vi "test TCX read (installed 71).vi"() -> ()   [LabVIEW 2011] (continued)
3:18:19Z</Time><Position><LatitudeDegrees>35.875570</LatitudeDegrees><LongitudeDegrees>-78.927722</LongitudeDegrees></Position><AltitudeMeters>68.872</AltitudeMeters><DistanceMeters>18272.553</DistanceMeters><Cadence>74</Cadence><Extensions><TPX xmlns=\"http://www.garmin.com/xmlschemas/ActivityExtension/v2\"><Watts>164</Watts></TPX></Extensions></Trackpoint><Trackpoint><Time>2008-03-03T23:18:20Z</Time><Position><LatitudeDegrees>35.875575</LatitudeDegrees><LongitudeDegrees>-78.927802</LongitudeDegrees></Position><AltitudeMeters>68.391</AltitudeMeters><DistanceMeters>18279.793</DistanceMeters><Cadence>73</Cadence><Extensions><TPX xmlns=\"http://www.garmin.com/xmlschemas/ActivityExtension/v2\"><Watts>157</Watts></TPX></Extensions></Trackpoint><Trackpoint><Time>2008-03-03T23:18:21Z</Time><Position><LatitudeDegrees>35.875583</LatitudeDegrees><LongitudeDegrees>-78.927883</LongitudeDegrees></Position><AltitudeMeters>68.872</AltitudeMeters><DistanceMeters>18287.141</DistanceMeters><Cadence>68</Cadence><Extensions><TPX xmlns=\"http://www.garmin.com/xmlschemas/ActivityExtension/v2\"><Watts>132</Watts></TPX></Extensions></Trackpoint><Trackpoint><Time>2008-03-03T23:18:22Z</Time><Position><LatitudeDegrees>35.875591</LatitudeDegrees><LongitudeDegrees>-78.927967</LongitudeDegrees></Position><AltitudeMeters>68.391</AltitudeMeters><DistanceMeters>18294.795</DistanceMeters><Cadence>69</Cadence><Extensions><TPX xmlns=\"http://www.garmin.com/xmlschemas/ActivityExtension/v2\"><Watts>106</Watts></TPX></Extensions></Trackpoint><Trackpoint><Time>2008-03-03T23:18:23Z</Time><Position><LatitudeDegrees>35.875599</LatitudeDegrees><LongitudeDegrees>-78.928051</LongitudeDegrees></Position><AltitudeMeters>68.872</AltitudeMeters><DistanceMeters>18302.459</DistanceMeters><Cadence>70</Cadence><Extensions><TPX xmlns=\"http://www.garmin.com/xmlschemas/ActivityExtension/v2\"><Watts>105</Watts></TPX></Extensions></Trackpoint><Trackpoint><Time>2008-03-03T23:18:24Z</Time><Position><LatitudeDegrees>35.875607</LatitudeDegrees><LongitudeDegrees>-78.928138</LongitudeDegrees></Position><AltitudeMeters>68.872</AltitudeMeters><DistanceMeters>18310.340</DistanceMeters><Cadence>71</Cadence><Extensions><TPX xmlns=\"http://www.garmin.com/xmlschemas/ActivityExtension/v2\"><Watts>95</Watts></TPX></Extensions></Trackpoint><Trackpoint><Time>2008-03-03T23:18:25Z</Time><Position><LatitudeDegrees>35.875615</LatitudeDegrees><LongitudeDegrees>-78.928227</LongitudeDegrees></Position><AltitudeMeters>68.391</AltitudeMeters><DistanceMeters>18318.404</DistanceMeters><Cadence>73</Cadence><Extensions><TPX xmlns=\"http://www.garmin.com/xmlschemas/ActivityExtension/v2\"><Watts>74</Watts></TPX></Extensions></Trackpoint><Trackpoint><Time>2008-03-03T23:18:26Z</Time><Position><LatitudeDegrees>35.875623</LatitudeDegrees><LongitudeDegrees>-78.928316</LongitudeDegrees></Position><AltitudeMeters>68.391</AltitudeMeters><DistanceMeters>18326.637</DistanceMeters><Cadence>75</Cadence><Extensions><TPX xmlns=\"http://www.garmin.com/xmlschemas/ActivityExtension/v2\"><Watts>63</Watts></TPX></Extensions></Trackpoint><Trackpoint><Time>2008-03-03T23:18:27Z</Time><Position><LatitudeDegrees>35.875631</LatitudeDegrees><LongitudeDegrees>-78.928409</LongitudeDegrees></Position><AltitudeMeters>67.910</AltitudeMeters><DistanceMeters>18334.977</DistanceMeters><Cadence>75</Cadence><Extensions><TPX xmlns=\"http://www.garmin.com/xmlschemas/ActivityExtension/v2\"><Watts>64</Watts></TPX></Extensions></Trackpoint><Trackpoint><Time>2008-03-03T23:18:28Z</Time><Position><LatitudeDegrees>35.875640</LatitudeDegrees><LongitudeDegrees>-78.928504</LongitudeDegrees></Position><AltitudeMeters>67.910</AltitudeMeters><DistanceMeters>18343.660</DistanceMeters><Cadence>81</Cadence><Extensions><TPX xmlns=\"http://www.garmin.com/xmlschemas/ActivityExtension/v2\"><Watts>53</Watts></TPX></Extensions></Trackpoint><Trackpoint><Time>2008-03-03T23:18:29Z</Time><Position><LatitudeDegrees>35.875651</LatitudeDegrees><LongitudeDegrees>-78.928603</LongitudeDegrees></Position><AltitudeMeters>67.910</AltitudeMeters><DistanceMeters>18352.664</DistanceMeters><Cadence>83</Cadence><Extensions><TPX xmlns=\"http://www.garmin.com/xmlschemas/ActivityExtension/v2\"><Watts>51</Watts></TPX></Extensions></Trackpoint><Trackpoint><Time>2008-03-03T23:18:30Z</Time><Position><LatitudeDegrees>35.875663</LatitudeDegrees><LongitudeDegrees>-78.928704</LongitudeDegrees></Position><AltitudeMeters>67.430</AltitudeMeters><DistanceMeters>18361.902</DistanceMeters><Cadence>85</Cadence><Extensions><TPX xmlns=\"http://www.garmin.com/xmlschemas/ActivityExtension/v2\"><Watts>48</Watts></TPX></Extensions></Trackpoint><Trackpoint><Time>2008-03-03T23:18:31Z</Time><Position><LatitudeDegrees>35.875675</LatitudeDegrees><LongitudeDegrees>-78.928807</LongitudeDegrees></Position><AltitudeMeters>66.949</AltitudeMeters><DistanceMeters>18371.299</DistanceMeters><Cadence>87</Cadence><Extensions><TPX xmlns=\"http://www.garmin.com/xmlschemas/ActivityExtension/v2\"><Watts>48</Watts></TPX></Extensions></Trackpoint><Trackpoint><Time>2008-03-03T23:18:32Z</Time><Position><LatitudeDegrees>35.875686</LatitudeDegrees><LongitudeDegrees>-78.928912</LongitudeDegrees></Position><AltitudeMeters>66.468</AltitudeMeters><DistanceMeters>18380.938</DistanceMeters><Cadence>90</Cadence><Extensions><TPX xmlns=\"http://www.garmin.com/xmlschemas/ActivityExtension/v2\"><Watts>50</Watts></TPX></Extensions></Trackpoint><Trackpoint><Time>2008-03-03T23:18:33Z</Time><Position><LatitudeDegrees>35.875695</LatitudeDegrees><LongitudeDegrees>-78.929021</LongitudeDegrees></Position><AltitudeMeters>65.988</AltitudeMeters><DistanceMeters>18390.785</DistanceMeters><Cadence>91</Cadence><Extensions><TPX xmlns=\"http://www.garmin.com/xmlschemas/ActivityExtension/v2\"><Watts>58</Watts></TPX></Extensions></Trackpoint><Trackpoint><Time>2008-03-03T23:18:34Z</Time><Position><LatitudeDegrees>35.875703</LatitudeDegrees><LongitudeDegrees>-78.929130</LongitudeDegrees></Position><AltitudeMeters>65.988</AltitudeMeters><DistanceMeters>18400.648</DistanceMeters><Cadence>91</Cadence><Extensions><TPX xmlns=\"http://www.garmin.com/xmlschemas/ActivityExtension/v2\"><Watts>66</Watts></TPX></Extensions></Trackpoint><Trackpoint><Time>2008-03-03T23:18:35Z</Time><Position><LatitudeDegrees>35.875709</LatitudeDegrees><LongitudeDegrees>-78.929239</LongitudeDegrees></Position><AltitudeMeters>65.988</AltitudeMeters><DistanceMeters>18410.574</DistanceMeters><Cadence>91</Cadence><Extensions><TPX xmlns=\"http://www.garmin.com/xmlschemas/ActivityExtension/v2\"><Watts>67</Watts></TPX></Extensions></Trackpoint><Trackpoint><Time>2008-03-03T23:18:36Z</Time><Position><LatitudeDegrees>35.875717</LatitudeDegrees><LongitudeDegrees>-78.929349</LongitudeDegrees></Position><AltitudeMeters>65.988</AltitudeMeters><DistanceMeters>18420.459</DistanceMeters><Cadence>91</Cadence><Extensions><TPX xmlns=\"http://www.garmin.com/xmlschemas/ActivityExtension/v2\"><Watts>71</Watts></TPX></Extensions></Trackpoint><Trackpoint><Time>2008-03-03T23:18:37Z</Time><Position><LatitudeDegrees>35.875727</LatitudeDegrees><LongitudeDegrees>-78.929458</LongitudeDegrees></Position><AltitudeMeters>65.988</AltitudeMeters><DistanceMeters>18430.391</DistanceMeters><Cadence>91</Cadence><Extensions><TPX xmlns=\"http://www.garmin.com/xmlschemas/ActivityExtension/v2\"><Watts>71</Watts></TPX></Extensions></Trackpoint><Trackpoint><Time>2008-03-03T23:18:38Z</Time><Position><LatitudeDegrees>35.875738</LatitudeDegrees><LongitudeDegrees>-78.929565</LongitudeDegrees></Position><AltitudeMeters>65.988</AltitudeMeters><DistanceMeters>18440.133</DistanceMeters><Cadence>90</Cadence><Extensions><TPX xmlns=\"http://www.garmin.com/xmlschemas/ActivityExtension/v2\"><Watts>78</Watts></TPX></Extensions></Trackpoint><Trackpoint><Time>2008-03-03T23:18:39Z</Time><Position><LatitudeDegrees>35.875745</LatitudeDegrees><LongitudeDegrees>-78.929673</LongitudeDegrees></Position><AltitudeMeters>65.507</AltitudeMeters><DistanceMeters>18449.887</DistanceMeters><Cadence>90</Cadence><Extensions><TPX xmlns=\"http://www.garmin.com/xmlschemas/ActivityExtension/v2\"><Watts>79</Watts></TPX></Extensions></Trackpoint><Trackpoint><Time>2008-03-03T23:18:40Z</Time><Position><LatitudeDegrees>35.875749</LatitudeDegrees><LongitudeDegrees>-78.929779</LongitudeDegrees></Position><AltitudeMeters>65.988</AltitudeMeters><DistanceMeters>18459.521</DistanceMeters><Cadence>89</Cadence><Extensions><TPX xmlns=\"http://www.garmin.com/xmlschemas/ActivityExtension/v2\"><Watts>101</Watts></TPX></Extensions></Trackpoint><Trackpoint><Time>2008-03-03T23:18:41Z</Time><Position><LatitudeDegrees>35.875754</LatitudeDegrees><LongitudeDegrees>-78.929886</LongitudeDegrees></Position><AltitudeMeters>65.988</AltitudeMeters><DistanceMeters>18469.232</DistanceMeters><Cadence>88</Cadence><Extensions><TPX xmlns=\"http://www.garmin.com/xmlschemas/ActivityExtension/v2\"><Watts>106</Watts></TPX></Extensions></Trackpoint><Trackpoint><Time>2008-03-03T23:18:42Z</Time><Position><LatitudeDegrees>35.875758</LatitudeDegrees><LongitudeDegrees>-78.929991</LongitudeDegrees></Position><AltitudeMeters>65.507</AltitudeMeters><DistanceMeters>18478.709</DistanceMeters><Cadence>87</Cadence><Extensions><TPX xmlns=\"http://www.garmin.com/xmlschemas/ActivityExtension/v2\"><Watts>106</Watts></TPX></Extensions></Trackpoint><Trackpoint><Time>2008-03-03T23:18:43Z</Time><Position><LatitudeDegrees>35.875761</LatitudeDegrees><LongitudeDegrees>-78.930095</LongitudeDegrees></Position><AltitudeMeters>65.507</AltitudeMeters><DistanceMeters>18488.055</DistanceMeters><Cadence>86</Cadence><Extensions><TPX xmlns=\"http://www.garmin.com/xmlschemas/ActivityExtension/v2\"><Watts>113</Watts></TPX></Extensions></Trackpoint><Trackpoint><Time>2008-03-03T23:18:44Z</Time><Position><LatitudeDegrees>35.875764</LatitudeDegrees><LongitudeDegrees>-78.930200</LongitudeDegrees></Position><AltitudeMeters>65.507</AltitudeMeters><DistanceMeters>18497.482</DistanceMeters><Cadence>86</Cadence><Extensions><TPX xmlns=\"http://www.garmin.com/xmlschemas/ActivityExtension/v2\"><Watts>112</Watts></TPX></Extensions></Trackpoint><Trackpoint><Time>2008-03-03T23:18:45Z</Time><Position><LatitudeDegrees>35.875767</LatitudeDegrees><LongitudeDegrees>-78.930301</LongitudeDegrees></Position><AltitudeMeters>65.507</AltitudeMeters><DistanceMeters>18506.688</DistanceMeters><Cadence>85</Cadence><Extensions><TPX xmlns=\"http://www.garmin.com/xmlschemas/ActivityExtension/v2\"><Watts>118</Watts></TPX></Extensions></Trackpoint><Trackpoint><Time>2008-03-03T23:18:46Z</Time><Position><LatitudeDegrees>35.875770</LatitudeDegrees><LongitudeDegrees>-78.930402</LongitudeDegrees></Position><AltitudeMeters>65.988</AltitudeMeters><DistanceMeters>18515.820</DistanceMeters><Cadence>84</Cadence><Extensions><TPX xmlns=\"http://www.garmin.com/xmlschemas/ActivityExtension/v2\"><Watts>133</Watts></TPX></Extensions></Trackpoint><Trackpoint><Time>2008-03-03T23:18:47Z</Time><Position><LatitudeDegrees>35.875772</LatitudeDegrees><LongitudeDegrees>-78.930502</LongitudeDegrees></Position><AltitudeMeters>65.988</AltitudeMeters><DistanceMeters>18524.832</DistanceMeters><Cadence>84</Cadence><Extensions><TPX xmlns=\"http://www.garmin.com/xmlschemas/ActivityExtension/v2\"><Watts>159</Watts></TPX></Extensions></Trackpoint><Trackpoint><Time>2008-03-03T23:18:48Z</Time><Position><LatitudeDegrees>35.875773</LatitudeDegrees><LongitudeDegrees>-78.930602</LongitudeDegrees></Position><AltitudeMeters>65.988</AltitudeMeters><DistanceMeters>18533.852</DistanceMeters><Cadence>83</Cadence><Extensions><TPX xmlns=\"http://www.garmin.com/xmlschemas/ActivityExtension/v2\"><Watts>166</Watts></TPX></Extensions></Trackpoint><Trackpoint><Time>2008-03-03T23:18:49Z</Time><Position><LatitudeDegrees>35.875777</LatitudeDegrees><LongitudeDegrees>-78.930701</LongitudeDegrees></Position><AltitudeMeters>65.988</AltitudeMeters><DistanceMeters>18542.797</DistanceMeters><Cadence>83</Cadence><Extensions><TPX xmlns=\"http://www.garmin.com/xmlschemas/ActivityExtension/v2\"><Watts>168</Watts></TPX></Extensions></Trackpoint><Trackpoint><Time>2008-03-03T23:18:50Z</Time><Position><LatitudeDegrees>35.875781</LatitudeDegrees><LongitudeDegrees>-78.930800</LongitudeDegrees></Position><AltitudeMeters>66.468</AltitudeMeters><DistanceMeters>18551.742</DistanceMeters><Cadence>82</Cadence><Extensions><TPX xmlns=\"http://www.garmin.com/xmlschemas/ActivityExtension/v2\"><Watts>183</Watts></TPX></Extensions></Trackpoint><Trackpoint><Time>2008-03-03T23:18:51Z</Time><Position><LatitudeDegrees>35.875783</LatitudeDegrees><LongitudeDegrees>-78.930898</LongitudeDegrees></Position><AltitudeMeters>65.988</AltitudeMeters><DistanceMeters>18560.613</DistanceMeters><Cadence>81</Cadence><Extensions><TPX xmlns=\"http://www.garmin.com/xmlschemas/ActivityExtension/v2\"><Watts>177</Watts></TPX></Extensions></Trackpoint><Trackpoint><Time>2008-03-03T23:18:52Z</Time><Position><LatitudeDegrees>35.875787</LatitudeDegrees><LongitudeDegrees>-78.930996</LongitudeDegrees></Position><AltitudeMeters>65.988</AltitudeMeters><DistanceMeters>18569.484</DistanceMeters><Cadence>80</Cadence><Extensions><TPX xmlns=\"http://www.garmin.com/xmlschemas/ActivityExtension/v2\"><Watts>171</Watts></TPX></Extensions></Trackpoint><Trackpoint><Time>2008-03-03T23:18:53Z</Time><Position><LatitudeDegrees>35.875790</LatitudeDegrees><LongitudeDegrees>-78.931093</LongitudeDegrees></Position><AltitudeMeters>65.988</AltitudeMeters><DistanceMeters>18578.180</DistanceMeters><Cadence>79</Cadence><Extensions><TPX xmlns=\"http://www.garmin.com/xmlschemas/ActivityExtension/v2\"><Watts>163</Watts></TPX></Extensions></Trackpoint><Trackpoint><Time>2008-03-03T23:18:54Z</Time><Position><LatitudeDegrees>35.875789</LatitudeDegrees><LongitudeDegrees>-78.931187</LongitudeDegrees></Position><AltitudeMeters>65.988</AltitudeMeters><DistanceMeters>18586.668</DistanceMeters><Cadence>79</Cadence><Extensions><TPX xmlns=\"http://www.garmin.com/xmlschemas/ActivityExtension/v2\"><Watts>162</Watts></TPX></Extensions></Trackpoint><Trackpoint><Time>2008-03-03T23:18:55Z</Time><Position><LatitudeDegrees>35.875786</LatitudeDegrees><LongitudeDegrees>-78.931280</LongitudeDegrees></Position><AltitudeMeters>65.988</AltitudeMeters><DistanceMeters>18595.109</DistanceMeters><Cadence>78</Cadence><Extensions><TPX xmlns=\"http://www.garmin.com/xmlschemas/ActivityExtension/v2\"><Watts>163</Watts></TPX></Extensions></Trackpoint><Trackpoint><Time>2008-03-03T23:18:56Z</Time><Position><LatitudeDegrees>35.875781</LatitudeDegrees><LongitudeDegrees>-78.931372</LongitudeDegrees></Position><AltitudeMeters>66.468</AltitudeMeters><DistanceMeters>18603.369</DistanceMeters><Cadence>77</Cadence><Extensions><TPX xmlns=\"http://www.garmin.com/xmlschemas/ActivityExtension/v2\"><Watts>164</Watts></TPX></Extensions></Trackpoint><Trackpoint><Time>2008-03-03T23:18:57Z</Time><Position><LatitudeDegrees>35.875773</LatitudeDegrees><LongitudeDegrees>-78.931461</LongitudeDegrees></Position><AltitudeMeters>66.468</AltitudeMeters><DistanceMeters>18611.516</DistanceMeters><Cadence>75</Cadence><Extensions><TPX xmlns=\"http://www.garmin.com/xmlschemas/ActivityExtension/v2\"><Watts>157</Watts></TPX></Extensions></Trackpoint><Trackpoint><Time>2008-03-03T23:18:58Z</Time><Position><LatitudeDegrees>35.875762</LatitudeDegrees><LongitudeDegrees>-78.931550</LongitudeDegrees></Position><AltitudeMeters>66.468</AltitudeMeters><DistanceMeters>18619.531</DistanceMeters><Cadence>73</Cadence><Extensions><TPX xmlns=\"http://www.garmin.com/xmlschemas/ActivityExtension/v2\"><Watts>164</Watts></TPX></Extensions></Trackpoint><Trackpoint><Time>2008-03-03T23:18:59Z</Time><Position><LatitudeDegrees>35.875749</LatitudeDegrees><LongitudeDegrees>-78.931636</LongitudeDegrees></Position><AltitudeMeters>66.949</AltitudeMeters><DistanceMeters>18627.453</DistanceMeters><Cadence>73</Cadence><Extensions><TPX xmlns=\"http://www.garmin.com/xmlschemas/ActivityExtension/v2\"><Watts>168</Watts></TPX></Extensions></Trackpoint><Trackpoint><Time>2008-03-03T23:19:00Z</Time><Position><LatitudeDegrees>35.875735</LatitudeDegrees><LongitudeDegrees>-78.931720</LongitudeDegrees></Position><AltitudeMeters>67.430</AltitudeMeters><DistanceMeters>18635.238</DistanceMeters><Cadence>71</Cadence><Extensions><TPX xmlns=\"http://www.garmin.com/xmlschemas/ActivityExtension/v2\"><Watts>181</Watts></TPX></Extensions></Trackpoint><Trackpoint><Time>2008-03-03T23:19:01Z</Time><Position><LatitudeDegrees>35.875721</LatitudeDegrees><LongitudeDegrees>-78.931803</LongitudeDegrees></Position><AltitudeMeters>67.430</AltitudeMeters><DistanceMeters>18642.844</DistanceMeters><Cadence>69</Cadence><Extensions><TPX xmlns=\"http://www.garmin.com/xmlschemas/ActivityExtension/v2\"><Watts>207</Watts></TPX></Extensions></Trackpoint><Trackpoint><Time>2008-03-03T23:19:02Z</Time><Position><LatitudeDegrees>35.875705</LatitudeDegrees><LongitudeDegrees>-78.931884</LongitudeDegrees></Position><AltitudeMeters>67.430</AltitudeMeters><DistanceMeters>18650.436</DistanceMeters><Cadence>70</Cadence><Extensions><TPX xmlns=\"http://www.garmin.com/xmlschemas/ActivityExtension/v2\"><Watts>205</Watts></TPX></Extensions></Trackpoint><Trackpoint><Time>2008-03-03T23:19:03Z</Time><Position><LatitudeDegrees>35.875691</LatitudeDegrees><LongitudeDegrees>-78.931962</LongitudeDegrees></Position><AltitudeMeters>67.910</AltitudeMeters><DistanceMeters>18657.533</DistanceMeters><Cadence>73</Cadence><Extensions><TPX xmlns=\"http://www.garmin.com/xmlschemas/ActivityExtension/v2\"><Watts>188</Watts></TPX></Extensions></Trackpoint><Trackpoint><Time>2008-03-03T23:19:04Z</Time><Position><LatitudeDegrees>35.875675</LatitudeDegrees><LongitudeDegrees>-78.932036</LongitudeDegrees></Position><AltitudeMeters>68.391</AltitudeMeters><DistanceMeters>18664.455</DistanceMeters><Cadence>73</Cadence><Extensions><TPX xmlns=\"http://www.garmin.com/xmlschemas/ActivityExtension/v2\"><Watts>185</Watts></TPX></Extensions></Trackpoint><Trackpoint><Time>2008-03-03T23:19:05Z</Time><Position><LatitudeDegrees>35.875659</LatitudeDegrees><LongitudeDegrees>-78.932107</LongitudeDegrees></Position><AltitudeMeters>68.391</AltitudeMeters><DistanceMeters>18671.105</DistanceMeters><Cadence>76</Cadence><Extensions><TPX xmlns=\"http://www.garmin.com/xmlschemas/ActivityExtension/v2\"><Watts>174</Watts></TPX></Extensions></Trackpoint><Trackpoint><Time>2008-03-03T23:19:06Z</Time><Position><LatitudeDegrees>35.875644</LatitudeDegrees><LongitudeDegrees>-78.932177</LongitudeDegrees></Position><AltitudeMeters>68.872</AltitudeMeters><DistanceMeters>18677.600</DistanceMeters><Cadence>78</Cadence><Extensions><TPX xmlns=\"http://www.garmin.com/xmlschemas/ActivityExtension/v2\"><Watts>173</Watts></TPX></Extensions></Trackpoint><Trackpoint><Time>2008-03-03T23:19:07Z</Time><Position><LatitudeDegrees>35.875631</LatitudeDegrees><LongitudeDegrees>-78.932247</LongitudeDegrees></Position><AltitudeMeters>69.352</AltitudeMeters><DistanceMeters>18684.131</DistanceMeters><Cadence>79</Cadence><Extensions><TPX xmlns=\"http://www.garmin.com/xmlschemas/ActivityExtension/v2\"><Watts>237</Watts></TPX></Extensions></Trackpoint><Trackpoint><Time>2008-03-03T23:19:08Z</Time><Position><LatitudeDegrees>35.875617</LatitudeDegrees><LongitudeDegrees>-78.932317</LongitudeDegrees></Position><AltitudeMeters>69.352</AltitudeMeters><DistanceMeters>18690.664</DistanceMeters><Cadence>79</Cadence><Extensions><TPX xmlns=\"http://www.garmin.com/xmlschemas/ActivityExtension/v2\"><Watts>338</Watts></TPX></Extensions></Trackpoint><Trackpoint><Time>2008-03-03T23:19:09Z</Time><Position><LatitudeDegrees>35.875603</LatitudeDegrees><LongitudeDegrees>-78.932388</LongitudeDegrees></Position><AltitudeMeters>69.833</AltitudeMeters><DistanceMeters>18697.219</DistanceMeters><Cadence>79</Cadence><Extensions><TPX xmlns=\"http://www.garmin.com/xmlschemas/ActivityExtension/v2\"><Watts>373</Watts></TPX></Extensions></Trackpoint><Trackpoint><Time>2008-03-03T23:19:10Z</Time><Position><LatitudeDegrees>35.875589</LatitudeDegrees><LongitudeDegrees>-78.932458</LongitudeDegrees></Position><AltitudeMeters>70.313</AltitudeMeters><DistanceMeters>18703.715</DistanceMeters><Cadence>78</Cadence><Extensions><TPX xmlns=\"http://www.garmin.com/xmlschemas/ActivityExtension/v2\"><Watts>371</Watts></TPX></Extensions></Trackpoint><Trackpoint><Time>2008-03-03T23:19:11Z</Time><Position><LatitudeDegrees>35.875575</LatitudeDegrees><LongitudeDegrees>-78.932527</LongitudeDegrees></Position><AltitudeMeters>70.794</AltitudeMeters><DistanceMeters>18710.178</DistanceMeters><Cadence>78</Cadence><Extensions><TPX xmlns=\"http://www.garmin.com/xmlschemas/ActivityExtension/v2\"><Watts>387</Watts></TPX></Extensions></Trackpoint><Trackpoint><Time>2008-03-03T23:19:12Z</Time><Position><LatitudeDegrees>35.875562</LatitudeDegrees><LongitudeDegrees>-78.932597</LongitudeDegrees></Position><AltitudeMeters>71.275</AltitudeMeters><DistanceMeters>18716.688</DistanceMeters><Cadence>79</Cadence><Extensions><TPX xmlns=\"http://www.garmin.com/xmlschemas/ActivityExtension/v2\"><Watts>457</Watts></TPX></Extensions></Trackpoint><Trackpoint><Time>2008-03-03T23:19:13Z</Time><Position><LatitudeDegrees>35.875548</LatitudeDegrees><LongitudeDegrees>-78.932668</LongitudeDegrees></Position><AltitudeMeters>71.755</AltitudeMeters><DistanceMeters>18723.232</DistanceMeters><Cadence>79</Cadence><Extensions><TPX xmlns=\"http://www.garmin.com/xmlschemas/ActivityExtension/v2\"><Watts>465</Watts></TPX></Extensions></Trackpoint><Trackpoint><Time>2008-03-03T23:19:14Z</Time><Position><LatitudeDegrees>35.875533</LatitudeDegrees><LongitudeDegrees>-78.932738</LongitudeDegrees></Position><AltitudeMeters>71.755</AltitudeMeters><DistanceMeters>18729.775</DistanceMeters><Cadence>79</Cadence><Extensions><TPX xmlns=\"http://www.garmin.com/xmlschemas/ActivityExtension/v2\"><Watts>467</Watts></TPX></Extensions></Trackpoint><Trackpoint><Time>2008-03-03T23:19:15Z</Time><Position><LatitudeDegrees>35.875519</LatitudeDegrees><LongitudeDegrees>-78.932808</LongitudeDegrees></Position><AltitudeMeters>72.236</AltitudeMeters><DistanceMeters>18736.256</DistanceMeters><Cadence>78</Cadence><Extensions><TPX xmlns=\"http://www.garmin.com/xmlschemas/ActivityExtension/v2\"><Watts>452</Watts></TPX></Extensions></Trackpoint><Trackpoint><Time>2008-03-03T23:19:16Z</Time><Position><LatitudeDegrees>35.875505</LatitudeDegrees><LongitudeDegrees>-78.932876</LongitudeDegrees></Position><AltitudeMeters>72.717</AltitudeMeters><DistanceMeters>18742.592</DistanceMeters><Cadence>78</Cadence><Extensions><TPX xmlns=\"http://www.garmin.com/xmlschemas/ActivityExtension/v2\"><Watts>448</Watts></TPX></Extensions></Trackpoint><Trackpoint><Time>2008-03-03T23:19:17Z</Time><Position><LatitudeDegrees>35.875492</LatitudeDegrees><LongitudeDegrees>-78.932942</LongitudeDegrees></Position><AltitudeMeters>73.198</AltitudeMeters><DistanceMeters>18748.783</DistanceMeters><Cadence>74</Cadence><Extensions><TPX xmlns=\"http://www.garmin.com/xmlschemas/ActivityExtension/v2\"><Watts>451</Watts></TPX></Extensions></Trackpoint><Trackpoint><Time>2008-03-03T23:19:18Z</Time><Position><LatitudeDegrees>35.875479</LatitudeDegrees><LongitudeDegrees>-78.933006</LongitudeDegrees></Position><AltitudeMeters>73.678</AltitudeMeters><DistanceMeters>18754.693</DistanceMeters><Cadence>71</Cadence><Extensions><TPX xmlns=\"http://www.garmin.com/xmlschemas/ActivityExtension/v2\"><Watts>459</Watts></TPX></Extensions></Trackpoint><Trackpoint><Time>2008-03-03T23:19:19Z</Time><Position><LatitudeDegrees>35.875466</LatitudeDegrees><LongitudeDegrees>-78.933069</LongitudeDegrees></Position><AltitudeMeters>73.678</AltitudeMeters><DistanceMeters>18760.582</DistanceMeters><Cadence>72</Cadence><Extensions><TPX xmlns=\"http://www.garmin.com/xmlschemas/ActivityExtension/v2\"><Watts>462</Watts></TPX></Extensions></Trackpoint><Trackpoint><Time>2008-03-03T23:19:20Z</Time><Position><LatitudeDegrees>35.875455</LatitudeDegrees><LongitudeDegrees>-78.933137</LongitudeDegrees></Position><AltitudeMeters>74.159</AltitudeMeters><DistanceMeters>18766.793</DistanceMeters><Cadence>73</Cadence><Extensions><TPX xmlns=\"http://www.garmin.com/xmlschemas/ActivityExtension/v2\"><Watts>525</Watts></TPX></Extensions></Trackpoint><Trackpoint><Time>2008-03-03T23:19:21Z</Time><Position><LatitudeDegrees>35.875441</LatitudeDegrees><LongitudeDegrees>-78.933206</LongitudeDegrees></Position><AltitudeMeters>74.640</AltitudeMeters><DistanceMeters>18773.268</DistanceMeters><Cadence>73</Cadence><Extensions><TPX xmlns=\"http://www.garmin.com/xmlschemas/ActivityExtension/v2\"><Watts>529</Watts></TPX></Extensions></Trackpoint><Trackpoint><Time>2008-03-03T23:19:22Z</Time><Position><LatitudeDegrees>35.875428</LatitudeDegrees><LongitudeDegrees>-78.933280</LongitudeDegrees></Position><AltitudeMeters>75.601</AltitudeMeters><DistanceMeters>18780.102</DistanceMeters><Cadence>83</Cadence><Extensions><TPX xmlns=\"http://www.garmin.com/xmlschemas/ActivityExtension/v2\"><Watts>697</Watts></TPX></Extensions></Trackpoint><Trackpoint><Time>2008-03-03T23:19:23Z</Time><Position><LatitudeDegrees>35.875415</LatitudeDegrees><LongitudeDegrees>-78.933356</LongitudeDegrees></Position><AltitudeMeters>75.601</AltitudeMeters><DistanceMeters>18787.135</DistanceMeters><Cadence>86</Cadence><Extensions><TPX xmlns=\"http://www.garmin.com/xmlschemas/ActivityExtension/v2\"><Watts>788</Watts></TPX></Extensions></Trackpoint><Trackpoint><Time>2008-03-03T23:19:24Z</Time><Position><LatitudeDegrees>35.875399</LatitudeDegrees><LongitudeDegrees>-78.933433</LongitudeDegrees></Position><AltitudeMeters>76.081</AltitudeMeters><DistanceMeters>18794.295</DistanceMeters><Cadence>86</Cadence><Extensions><TPX xmlns=\"http://www.garmin.com/xmlschemas/ActivityExtension/v2\"><Watts>782</Watts></TPX></Extensions></Trackpoint><Trackpoint><Time>2008-03-03T23:19:25Z</Time><Position><LatitudeDegrees>35.875377</LatitudeDegrees><LongitudeDegrees>-78.933509</LongitudeDegrees></Position><AltitudeMeters>77.043</AltitudeMeters><DistanceMeters>18801.568</DistanceMeters><Cadence>89</Cadence><Extensions><TPX xmlns=\"http://www.garmin.com/xmlschemas/ActivityExtension/v2\"><Watts>738</Watts></TPX></Extensions></Trackpoint><Trackpoint><Time>2008-03-03T23:19:26Z</Time><Position><LatitudeDegrees>35.875358</LatitudeDegrees><LongitudeDegrees>-78.933588</LongitudeDegrees></Position><AltitudeMeters>77.043</AltitudeMeters><DistanceMeters>18809.012</DistanceMeters><Cadence>91</Cadence><Extensions><TPX xmlns=\"http://www.garmin.com/xmlschemas/ActivityExtension/v2\"><Watts>743</Watts></TPX></Extensions></Trackpoint><Trackpoint><Time>2008-03-03T23:19:27Z</Time><Position><LatitudeDegrees>35.875341</LatitudeDegrees><LongitudeDegrees>-78.933670</LongitudeDegrees></Position><AltitudeMeters>77.523</AltitudeMeters><DistanceMeters>18816.676</DistanceMeters><Cadence>92</Cadence><Extensions><TPX xmlns=\"http://www.garmin.com/xmlschemas/ActivityExtension/v2\"><Watts>701</Watts></TPX></Extensions></Trackpoint><Trackpoint><Time>2008-03-03T23:19:28Z</Time><Position><LatitudeDegrees>35.875323</LatitudeDegrees><LongitudeDegrees>-78.933751</LongitudeDegrees></Position><AltitudeMeters>78.485</AltitudeMeters><DistanceMeters>18824.240</DistanceMeters><Cadence>91</Cadence><Extensions><TPX xmlns=\"http://www.garmin.com/xmlschemas/ActivityExtension/v2\"><Watts>567</Watts></TPX></Extensions></Trackpoint><Trackpoint><Time>2008-03-03T23:19:29Z</Time><Position><LatitudeDegrees>35.875308</LatitudeDegrees><LongitudeDegrees>-78.933832</LongitudeDegrees></Position><AltitudeMeters>79.446</AltitudeMeters><DistanceMeters>18831.688</DistanceMeters><Cadence>89</Cadence><Extensions><TPX xmlns=\"http://www.garmin.com/xmlschemas/ActivityExtension/v2\"><Watts>466</Watts></TPX></Extensions></Trackpoint><Trackpoint><Time>2008-03-03T23:19:30Z</Time><Position><LatitudeDegrees>35.875294</LatitudeDegrees><LongitudeDegrees>-78.933909</LongitudeDegrees></Position><AltitudeMeters>80.407</AltitudeMeters><DistanceMeters>18838.797</DistanceMeters><Cadence>82</Cadence><Extensions><TPX xmlns=\"http://www.garmin.com/xmlschemas/ActivityExtension/v2\"><Watts>351</Watts></TPX></Extensions></Trackpoint><Trackpoint><Time>2008-03-03T23:19:31Z</Time><Position><LatitudeDegrees>35.875281</LatitudeDegrees><LongitudeDegrees>-78.933981</LongitudeDegrees></Position><AltitudeMeters>80.407</AltitudeMeters><DistanceMeters>18845.441</DistanceMeters><Cadence>82</Cadence><Extensions><TPX xmlns=\"http://www.garmin.com/xmlschemas/ActivityExtension/v2\"><Watts>353</Watts></TPX></Extensions></Trackpoint><Trackpoint><Time>2008-03-03T23:19:32Z</Time><Position><LatitudeDegrees>35.875268</LatitudeDegrees><LongitudeDegrees>-78.934050</LongitudeDegrees></Position><AltitudeMeters>80.888</AltitudeMeters><DistanceMeters>18851.893</DistanceMeters><Cadence>76</Cadence><Extensions><TPX xmlns=\"http://www.garmin.com/xmlschemas/ActivityExtension/v2\"><Watts>249</Watts></TPX></Extensions></Trackpoint><Trackpoint><Time>2008-03-03T23:19:33Z</Time><Position><LatitudeDegrees>35.875255</LatitudeDegrees><LongitudeDegrees>-78.934119</LongitudeDegrees></Position><AltitudeMeters>81.369</AltitudeMeters><DistanceMeters>18858.248</DistanceMeters><Cadence>76</Cadence><Extensions><TPX xmlns=\"http://www.garmin.com/xmlschemas/ActivityExtension/v2\"><Watts>248</Watts></TPX></Extensions></Trackpoint><Trackpoint><Time>2008-03-03T23:19:34Z</Time><Position><LatitudeDegrees>35.875243</LatitudeDegrees><LongitudeDegrees>-78.934186</LongitudeDegrees></Position><AltitudeMeters>81.369</AltitudeMeters><DistanceMeters>18864.459</DistanceMeters><Cadence>75</Cadence><Extensions><TPX xmlns=\"http://www.garmin.com/xmlschemas/ActivityExtension/v2\"><Watts>240</Watts></TPX></Extensions></Trackpoint><Trackpoint><Time>2008-03-03T23:19:35Z</Time><Position><LatitudeDegrees>35.875231</LatitudeDegrees><LongitudeDegrees>-78.934252</LongitudeDegrees></Position><AltitudeMeters>81.369</AltitudeMeters><DistanceMeters>18870.562</DistanceMeters><Cadence>73</Cadence><Extensions><TPX xmlns=\"http://www.garmin.com/xmlschemas/ActivityExtension/v2\"><Watts>241</Watts></TPX></Extensions></Trackpoint><Trackpoint><Time>2008-03-03T23:19:36Z</Time><Position><LatitudeDegrees>35.875217</LatitudeDegrees><LongitudeDegrees>-78.934317</LongitudeDegrees></Position><AltitudeMeters>81.849</AltitudeMeters><DistanceMeters>18876.643</DistanceMeters><Cadence>72</Cadence><Extensions><TPX xmlns=\"http://www.garmin.com/xmlschemas/ActivityExtension/v2\"><Watts>250</Watts></TPX></Extensions></Trackpoint><Trackpoint><Time>2008-03-03T23:19:37Z</Time><Position><LatitudeDegrees>35.875204</LatitudeDegrees><LongitudeDegrees>-78.934383</LongitudeDegrees></Position><AltitudeMeters>81.849</AltitudeMeters><DistanceMeters>18882.711</DistanceMeters><Cadence>73</Cadence><Extensions><TPX xmlns=\"http://www.garmin.com/xmlschemas/ActivityExtension/v2\"><Watts>229</Watts></TPX></Extensions></Trackpoint><Trackpoint><Time>2008-03-03T23:19:38Z</Time><Position><LatitudeDegrees>35.875192</LatitudeDegrees><LongitudeDegrees>-78.934448</LongitudeDegrees></Position><AltitudeMeters>81.849</AltitudeMeters><DistanceMeters>18888.758</DistanceMeters><Cadence>73</Cadence><Extensions><TPX xmlns=\"http://www.garmin.com/xmlschemas/ActivityExtension/v2\"><Watts>223</Watts></TPX></Extensions></Trackpoint><Trackpoint><Time>2008-03-03T23:19:39Z</Time><Position><LatitudeDegrees>35.875180</LatitudeDegrees><LongitudeDegrees>-78.934514</LongitudeDegrees></Position><AltitudeMeters>81.849</AltitudeMeters><DistanceMeters>18894.848</DistanceMeters><Cadence>73</Cadence><Extensions><TPX xmlns=\"http://www.garmin.com/xmlschemas/ActivityExtension/v2\"><Watts>210</Watts></TPX></Extensions></Trackpoint><Trackpoint><Time>2008-03-03T23:19:40Z</Time><Position><LatitudeDegrees>35.875167</LatitudeDegrees><LongitudeDegrees>-78.934579</LongitudeDegrees></Position><AltitudeMeters>82.330</AltitudeMeters><DistanceMeters>18900.934</DistanceMeters><Cadence>73</Cadence><Extensions><TPX xmlns=\"http://www.garmin.com/xmlschemas/ActivityExtension/v2\"><Watts>205</Watts></TPX></Extensions></Trackpoint><Trackpoint><Time>2008-03-03T23:19:41Z</Time><Position><LatitudeDegrees>35.875155</LatitudeDegrees><LongitudeDegrees>-78.934645</LongitudeDegrees></Position><AltitudeMeters>82.811</AltitudeMeters><DistanceMeters>18907.023</DistanceMeters><Cadence>73</Cadence><Extensions><TPX xmlns=\"http://www.garmin.com/xmlschemas/ActivityExtension/v2\"><Watts>202</Watts></TPX></Extensions></Trackpoint><Trackpoint><Time>2008-03-03T23:19:42Z</Time><Position><LatitudeDegrees>35.875144</LatitudeDegrees><LongitudeDegrees>-78.934711</LongitudeDegrees></Position><AltitudeMeters>82.811</AltitudeMeters><DistanceMeters>18913.080</DistanceMeters><Cadence>72</Cadence><Extensions><TPX xmlns=\"http://www.garmin.com/xmlschemas/ActivityExtension/v2\"><Watts>175</Watts></TPX></Extensions></Trackpoint><Trackpoint><Time>2008-03-03T23:19:43Z</Time><Position><LatitudeDegrees>35.875132</LatitudeDegrees><LongitudeDegrees>-78.934777</LongitudeDegrees></Position><AltitudeMeters>82.811</AltitudeMeters><DistanceMeters>18919.154</DistanceMeters><Cadence>72</Cadence><Extensions><TPX xmlns=\"http://www.garmin.com/xmlschemas/ActivityExtension/v2\"><Watts>175</Watts></TPX></Extensions></Trackpoint><Trackpoint><Time>2008-03-03T23:19:44Z</Time><Position><LatitudeDegrees>35.875120</LatitudeDegrees><LongitudeDegrees>-78.934843</LongitudeDegrees></Position><AltitudeMeters>82.811</AltitudeMeters><DistanceMeters>18925.324</DistanceMeters><Cadence>73</Cadence><Extensions><TPX xmlns=\"http://www.garmin.com/xmlschemas/ActivityExtension/v2\"><Watts>173</Watts></TPX></Extensions></Trackpoint><Trackpoint><Time>2008-03-03T23:19:45Z</Time><Position><LatitudeDegrees>35.875105</LatitudeDegrees><LongitudeDegrees>-78.934909</LongitudeDegrees></Position><AltitudeMeters>82.811</AltitudeMeters><DistanceMeters>18931.518</DistanceMeters><Cadence>75</Cadence><Extensions><TPX xmlns=\"http://www.garmin.com/xmlschemas/ActivityExtension/v2\"><Watts>173</Watts></TPX></Extensions></Trackpoint><Trackpoint><Time>2008-03-03T23:19:46Z</Time><Position><LatitudeDegrees>35.875092</LatitudeDegrees><LongitudeDegrees>-78.934976</LongitudeDegrees></Position><AltitudeMeters>82.811</AltitudeMeters><DistanceMeters>18937.707</DistanceMeters><Cadence>75</Cadence><Extensions><TPX xmlns=\"http://www.garmin.com/xmlschemas/ActivityExtension/v2\"><Watts>157</Watts></TPX></Extensions></Trackpoint><Trackpoint><Time>2008-03-03T23:19:47Z</Time><Position><LatitudeDegrees>35.875078</LatitudeDegrees><LongitudeDegrees>-78.935043</LongitudeDegrees></Position><AltitudeMeters>82.811</AltitudeMeters><DistanceMeters>18943.947</DistanceMeters><Cadence>75</Cadence><Extensions><TPX xmlns=\"http://www.garmin.com/xmlschemas/ActivityExtension/v2\"><Watts>138</Watts></TPX></Extensions></Trackpoint><Trackpoint><Time>2008-03-03T23:19:48Z</Time><Position><LatitudeDegrees>35.875064</LatitudeDegrees><LongitudeDegrees>-78.935111</LongitudeDegrees></Position><AltitudeMeters>83.291</AltitudeMeters><DistanceMeters>18950.324</DistanceMeters><Cadence>76</Cadence><Extensions><TPX xmlns=\"http://www.garmin.com/xmlschemas/ActivityExtension/v2\"><Watts>133</Watts></TPX></Extensions></Trackpoint><Trackpoint><Time>2008-03-03T23:19:49Z</Time><Position><LatitudeDegrees>35.875050</LatitudeDegrees><LongitudeDegrees>-78.935181</LongitudeDegrees></Position><AltitudeMeters>83.291</AltitudeMeters><DistanceMeters>18956.779</DistanceMeters><Cadence>78</Cadence><Extensions><TPX xmlns=\"http://www.garmin.com/xmlschemas/ActivityExtension/v2\"><Watts>133</Watts></TPX></Extensions></Trackpoint><Trackpoint><Time>2008-03-03T23:19:50Z</Time><Position><LatitudeDegrees>35.875038</LatitudeDegrees><LongitudeDegrees>-78.935251</LongitudeDegrees></Position><AltitudeMeters>82.811</AltitudeMeters><DistanceMeters>18963.340</DistanceMeters><Cadence>79</Cadence><Extensions><TPX xmlns=\"http://www.garmin.com/xmlschemas/ActivityExtension/v2\"><Watts>117</Watts></TPX></Extensions></Trackpoint><Trackpoint><Time>2008-03-03T23:19:51Z</Time><Position><LatitudeDegrees>35.875024</LatitudeDegrees><LongitudeDegrees>-78.935322</LongitudeDegrees></Position><AltitudeMeters>83.291</AltitudeMeters><DistanceMeters>18969.873</DistanceMeters><Cadence>79</Cadence><Extensions><TPX xmlns=\"http://www.garmin.com/xmlschemas/ActivityExtension/v2\"><Watts>120</Watts></TPX></Extensions></Trackpoint><Trackpoint><Time>2008-03-03T23:19:52Z</Time><Position><LatitudeDegrees>35.875010</LatitudeDegrees><LongitudeDegrees>-78.935394</LongitudeDegrees></Position><AltitudeMeters>83.291</AltitudeMeters><DistanceMeters>18976.574</DistanceMeters><Cadence>81</Cadence><Extensions><TPX xmlns=\"http://www.garmin.com/xmlschemas/ActivityExtension/v2\"><Watts>85</Watts></TPX></Extensions></Trackpoint><Trackpoint><Time>2008-03-03T23:19:53Z</Time><Position><LatitudeDegrees>35.874995</LatitudeDegrees><LongitudeDegrees>-78.935466</LongitudeDegrees></Position><AltitudeMeters>83.291</AltitudeMeters><DistanceMeters>18983.314</DistanceMeters><Cadence>81</Cadence><Extensions><TPX xmlns=\"http://www.garmin.com/xmlschemas/ActivityExtension/v2\"><Watts>86</Watts></TPX></Extensions></Trackpoint><Trackpoint><Time>2008-03-03T23:19:54Z</Time><Position><LatitudeDegrees>35.874981</LatitudeDegrees><LongitudeDegrees>-78.935539</LongitudeDegrees></Position><AltitudeMeters>83.291</AltitudeMeters><DistanceMeters>18990.107</DistanceMeters><Cadence>81</Cadence><Extensions><TPX xmlns=\"http://www.garmin.com/xmlschemas/ActivityExtension/v2\"><Watts>86</Watts></TPX></Extensions></Trackpoint><Trackpoint><Time>2008-03-03T23:19:55Z</Time><Position><LatitudeDegrees>35.874967</LatitudeDegrees><LongitudeDegrees>-78.935613</LongitudeDegrees></Position><AltitudeMeters>83.291</AltitudeMeters><DistanceMeters>18996.941</DistanceMeters><Cadence>82</Cadence><Extensions><TPX xmlns=\"http://www.garmin.com/xmlschemas/ActivityExtension/v2\"><Watts>88</Watts></TPX></Extensions></Trackpoint><Trackpoint><Time>2008-03-03T23:19:56Z</Time><Position><LatitudeDegrees>35.874953</LatitudeDegrees><LongitudeDegrees>-78.935687</LongitudeDegrees></Position><AltitudeMeters>83.291</AltitudeMeters><DistanceMeters>19003.799</DistanceMeters><Cadence>82</Cadence><Extensions><TPX xmlns=\"http://www.garmin.com/xmlschemas/ActivityExtension/v2\"><Watts>88</Watts></TPX></Extensions></Trackpoint><Trackpoint><Time>2008-03-03T23:19:57Z</Time><Position><LatitudeDegrees>35.874942</LatitudeDegrees><LongitudeDegrees>-78.935761</LongitudeDegrees></Position><AltitudeMeters>83.291</AltitudeMeters><DistanceMeters>19010.586</DistanceMeters><Cadence>82</Cadence><Extensions><TPX xmlns=\"http://www.garmin.com/xmlschemas/ActivityExtension/v2\"><Watts>94</Watts></TPX></Extensions></Trackpoint><Trackpoint><Time>2008-03-03T23:19:58Z</Time><Position><LatitudeDegrees>35.874931</LatitudeDegrees><LongitudeDegrees>-78.935836</LongitudeDegrees></Position><AltitudeMeters>83.291</AltitudeMeters><DistanceMeters>19017.412</DistanceMeters><Cadence>82</Cadence><Extensions><TPX xmlns=\"http://www.garmin.com/xmlschemas/ActivityExtension/v2\"><Watts>93</Watts></TPX></Extensions></Trackpoint><Trackpoint><Time>2008-03-03T23:19:59Z</Time><Position><LatitudeDegrees>35.874921</LatitudeDegrees><LongitudeDegrees>-78.935911</LongitudeDegrees></Position><AltitudeMeters>83.291</AltitudeMeters><DistanceMeters>19024.318</DistanceMeters><Cadence>83</Cadence><Extensions><TPX xmlns=\"http://www.garmin.com/xmlschemas/ActivityExtension/v2\"><Watts>105</Watts></TPX></Extensions></Trackpoint><Trackpoint><Time>2008-03-03T23:20:00Z</Time><Position><LatitudeDegrees>35.874913</LatitudeDegrees><LongitudeDegrees>-78.935986</LongitudeDegrees></Position><AltitudeMeters>83.772</AltitudeMeters><DistanceMeters>19031.195</DistanceMeters><Cadence>81</Cadence><Extensions><TPX xmlns=\"http://www.garmin.com/xmlschemas/ActivityExtension/v2\"><Watts>105</Watts></TPX></Extensions></Trackpoint><Trackpoint><Time>2008-03-03T23:20:01Z</Time><Position><LatitudeDegrees>35.874907</LatitudeDegrees><LongitudeDegrees>-78.936061</LongitudeDegrees></Position><AltitudeMeters>83.772</AltitudeMeters><DistanceMeters>19037.975</DistanceMeters><Cadence>80</Cadence><Extensions><TPX 
